vi "TS Next State.vi"(10 "Next State?":bool, 11 "Array in":T1[](array[typedef])) -> (3 "Array out":T1[](array[typedef]))   [LabVIEW 2017]
uses:
  controls/Test Sequencer.ctl
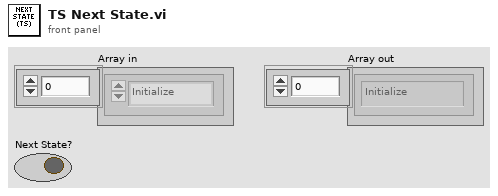
[diagram p1: front panel]
types:
  T1 = typedef "Test Sequencer.ctl" = enum16{"Initialize", "Clamp", "Homing (DOWN)", "Go Up", "Go DOWN", "Go UP (Loaded)", "Stall Force", "Go DOWN (Loaded)", "Shipping Position", "De-Clamp", "Result Checker"}
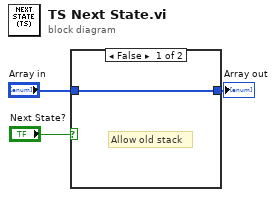
[diagram p0: block diagram]
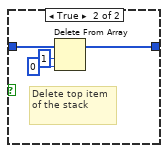
[diagram p2: hidden frame]
diagram:
  n1 = case shown="False" "Next State?" {
    tunnel: [w4 w6] -> w1
    tunnel: "Array in" -> [w4 w5]
    frame False {
      # "Allow old stack"
    }
    frame True {
      # "Delete top item of the stack"
      n2 = Delete From Array(array=w5, length=1, index=0) -> (array with subset deleted=w6:T1[])  [unwired: 1 out]
    }
  }
  "Array out" <- w1
